vi "REPORT_PACE_recolor_columns.vi"(6 "Recolor? (T)":bool=TRUE, 8 "error_in":errorcluster, 10 "records":string[][](array[string]), 11 "listbox_ref":refnum<vi>) -> (0 "error_out":errorcluster)   [LabVIEW 2019]
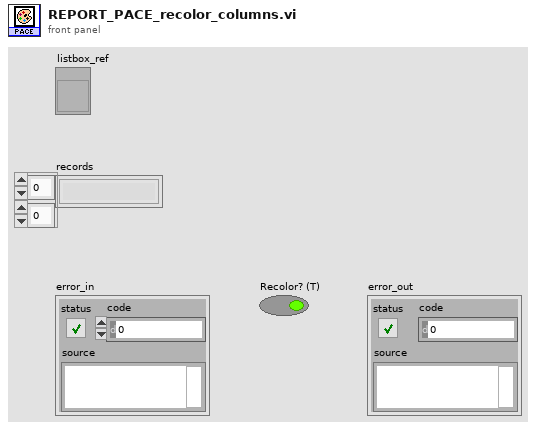
[diagram p1: front panel]
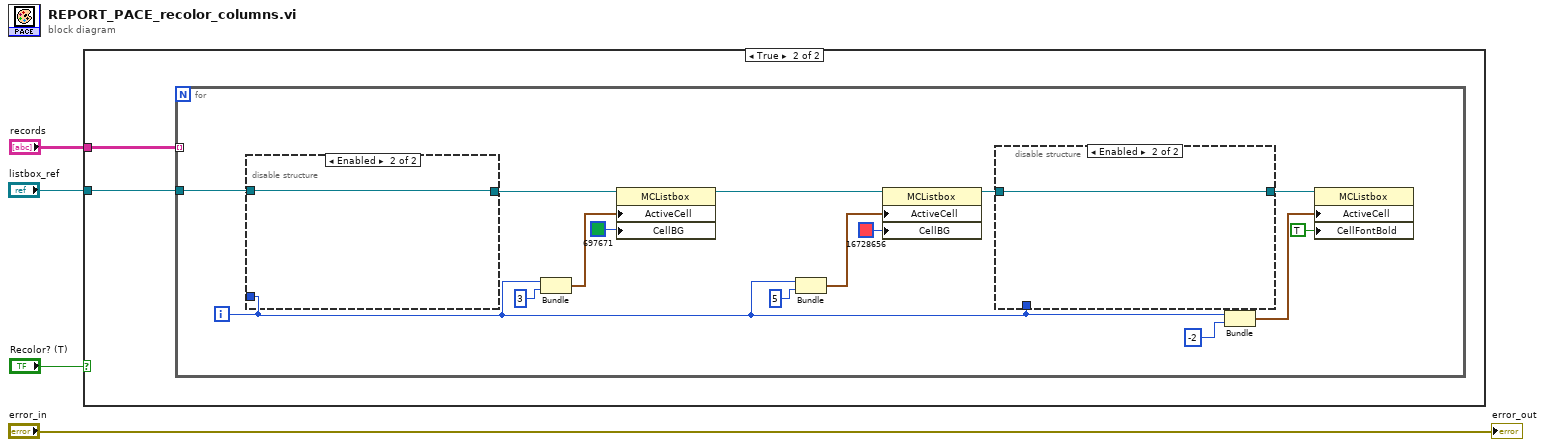
[diagram p0: block diagram]
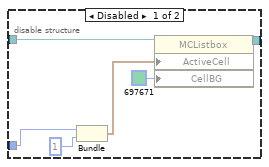
[diagram p3: hidden frame]
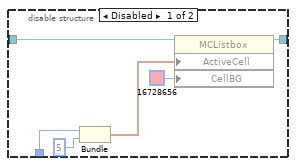
[diagram p4: hidden frame]
diagram:
  n1 = case shown="True" "Recolor? (T)" {
    tunnel: "records" -> [_ w5]
    tunnel: "listbox_ref" -> [_ w6]
    frame False {
    }
    frame True {
      n2 = for {
        tunnel: w6 -> [w21]
        tunnel: w5 -> [_] mode=indexing
        i -> [w8]
        n3 = disable-structure shown="Enabled" {
          disable-tunnel: w21 -> [w27 w28]
          disable-tunnel: [w24 w28] -> w20
          disable-tunnel: w8 -> [w22 _]
          frame Disabled {
            n4 = Bundle(w22, 1) -> (w25:cluster{i32, i32})  [unwired: 1 in]
            n5 = property on="Property Node" class="MCListbox"(reference=w27, "ActiveCell"=w25, "CellBG"=u32 697671) -> (reference out=w24:refnum<vi>)  [unwired: 1 in, 1 out]
          }
          frame Enabled {
          }
        }
        n6 = Bundle(w8, 3) -> (w11:cluster{i32, i32})  [unwired: 1 in]
        n7 = property on="Property Node" class="MCListbox"(reference=w20, "ActiveCell"=w11, "CellBG"=u32 697671) -> (reference out=w16:refnum<vi>)  [unwired: 1 in, 1 out]
        n8 = Bundle(w8, 5) -> (w7:cluster{i32, i32})  [unwired: 1 in]
        n9 = property on="Property Node" class="MCListbox"(reference=w16, "ActiveCell"=w7, "CellBG"=u32 16728656) -> (reference out=w15:refnum<vi>)  [unwired: 1 in, 1 out]
        n10 = disable-structure shown="Enabled" {
          disable-tunnel: w15 -> [w34 w35]
          disable-tunnel: [w33 w35] -> w14
          disable-tunnel: w8 -> [w30 _]
          frame Disabled {
            n11 = Bundle(w30, 5) -> (w29:cluster{i32, i32})  [unwired: 1 in]
            n12 = property on="Property Node" class="MCListbox"(reference=w34, "ActiveCell"=w29, "CellBG"=u32 16728656) -> (reference out=w33:refnum<vi>)  [unwired: 1 in, 1 out]
          }
          frame Enabled {
          }
        }
        n13 = Bundle(w8, -2) -> (w18:cluster{i32, i32})  [unwired: 1 in]
        n14 = property on="Property Node" class="MCListbox"(reference=w14, "ActiveCell"=w18, "CellFontBold"=TRUE ("Active Cell:Cell Font:Bold")) -> ()  [unwired: 1 in, 2 out]
      }
    }
  }
  "error_out" <- "error_in"
